vi "RemoveVersionsPoints.vi"(11 "Version 1":string) -> (3 "result string":string)   [LabVIEW 2019, in "ByteLVDevEnv.lvlib"]
uses:
  ByteLVDevEnv.lvlib
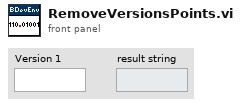
[diagram p1: front panel]
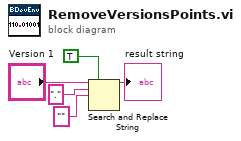
[diagram p0: block diagram]
diagram:
  n1 = Search and Replace String(replace all?=TRUE ("replace all? (F)"), input string="Version 1", search string=".", replace string="" ("replace string (\"\")")) -> (result string=→"result string":string)  [unwired: 4 in, 3 out]
